vi "Set Temperature Event.vi"(8 "error in (no error)":errorcluster, 11 "temperatureEvent":u32) -> (0 "error out":errorcluster, 2 "function return":u32, 3 "temperatureEvent out":u32)   [LabVIEW 2014, in "atmcd32d.lvlib"]
doc: "unsigned int WINAPI SetTemperatureEvent(HANDLE temperatureEvent);"
uses:
  atmcd32d.lvlib
  atmcd32d.dll
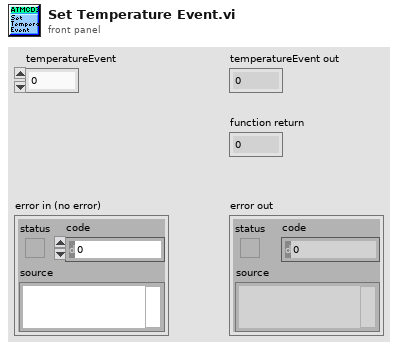
[diagram p1: front panel]
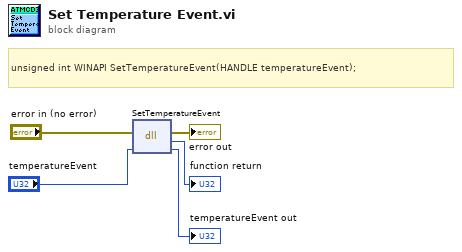
[diagram p0: block diagram]
diagram:
  # "unsigned int WINAPI SetTemperatureEvent(HANDLE temperatureEvent);"
  n1 = dll-call lib="C:/Users/Bakir/Documents/Lambda2-Testing/lib/Andorlib/atmcd32d.*" fn="SetTemperatureEvent"(error in="error in (no error)", "temperatureEvent"="temperatureEvent") -> (error out=→"error out":errorcluster, →"function return":u32, "temperatureEvent"=→"temperatureEvent out":u32)  [unwired: 2 in, 1 out]
